vi "FindPosForItem.vi"(0 "reference in":refnum<class "DQMHModuleNode.lvclass">, 1 "SearchItem":string, 2 "AttributesIDs":string[](array[string]), 3 "MethodIDs":string[](array[string]), 5 "error in (no error)":errorcluster) -> (12 "UpperRightPoint":T1 {"y" format="%.2f"; "x" format="%.2f"}, 14 "reference out":refnum<class "DQMHModuleNode.lvclass">, 15 "LeftPoint":T1 {"y" format="%.2f"; "x" format="%.2f"}, 16 "CenterPoint":T1 {"y" format="%.2f"; "x" format="%.2f"}, 17 "RightPoint":T1 {"y" format="%.2f"; "x" format="%.2f"}, 18 "UpperLeftPoint":T1 {"y" format="%.2f"; "x" format="%.2f"}, 19 "error out":errorcluster)   [LabVIEW 2020, in "DQMHModuleNode.lvclass"]
doc: "public void draw(Graphics2D g2, Point2D p, Point2D q)"
uses:
  <resource>/Framework/Providers/Open_GDS/UML/DQMHModuleNode_class/DQMHModuleNode.lvclass
  C:/Program Files (x86)/National Instruments/LabVIEW 2020/resource/Framework/Providers/Open_GDS/UML/RectangularNode_class/RectangularNode.lvclass
  <resource>/Framework/Providers/Open_GDS/UML/General/Point/Point Point2D.ctl
  <resource>/Framework/Providers/Open_GDS/UML/General/Rectangle/Rectangle Rectangle2D.ctl
  <resource>/Framework/Providers/Open_GDS/UML/MultiLineString_class/MultiLineString.lvclass
  <resource>/Framework/Providers/Open_GDS/UML/RectangularNode_class/RectangularNode.lvclass
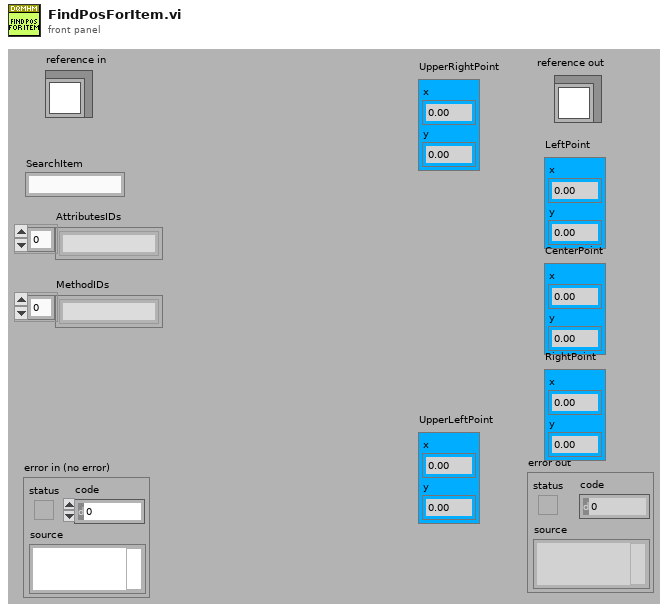
[diagram p1: front panel]
types:
  T1 = typedef "Point Point2D.ctl" = cluster{"x":dbl, "y":dbl}
  T2 = typedef "Rectangle Rectangle2D.ctl" = cluster{"x":dbl, "y":dbl, "width":dbl, "height":dbl}
  T3 = typedef "DQMHModuleNode.lvclass/ObjectAttributes.ctl" = cluster{"DescriptionHeight":dbl, "InternalDataHeight":dbl, "EventsHeight":dbl, "Name":refnum<class "MultiLineString.lvclass">, "Description":refnum<class "MultiLineString.lvclass">, "InternalData":refnum<class "MultiLineString.lvclass">, "Events":refnum<class "MultiLineString.lvclass">, "showDescription":bool, "showInternalData":bool, "showEvents":bool, "DEFAULT_ROUNDING":i32, "DEFAULT_WIDTH":i32, "DEFAULT_HEIGHT":i32, "ClassPath":path, "Template":string, "Icon":u8[][]}
  T4 = typedef "RectangularNode.lvclass/ObjectAttributes.ctl" = cluster{"bounds":T2}
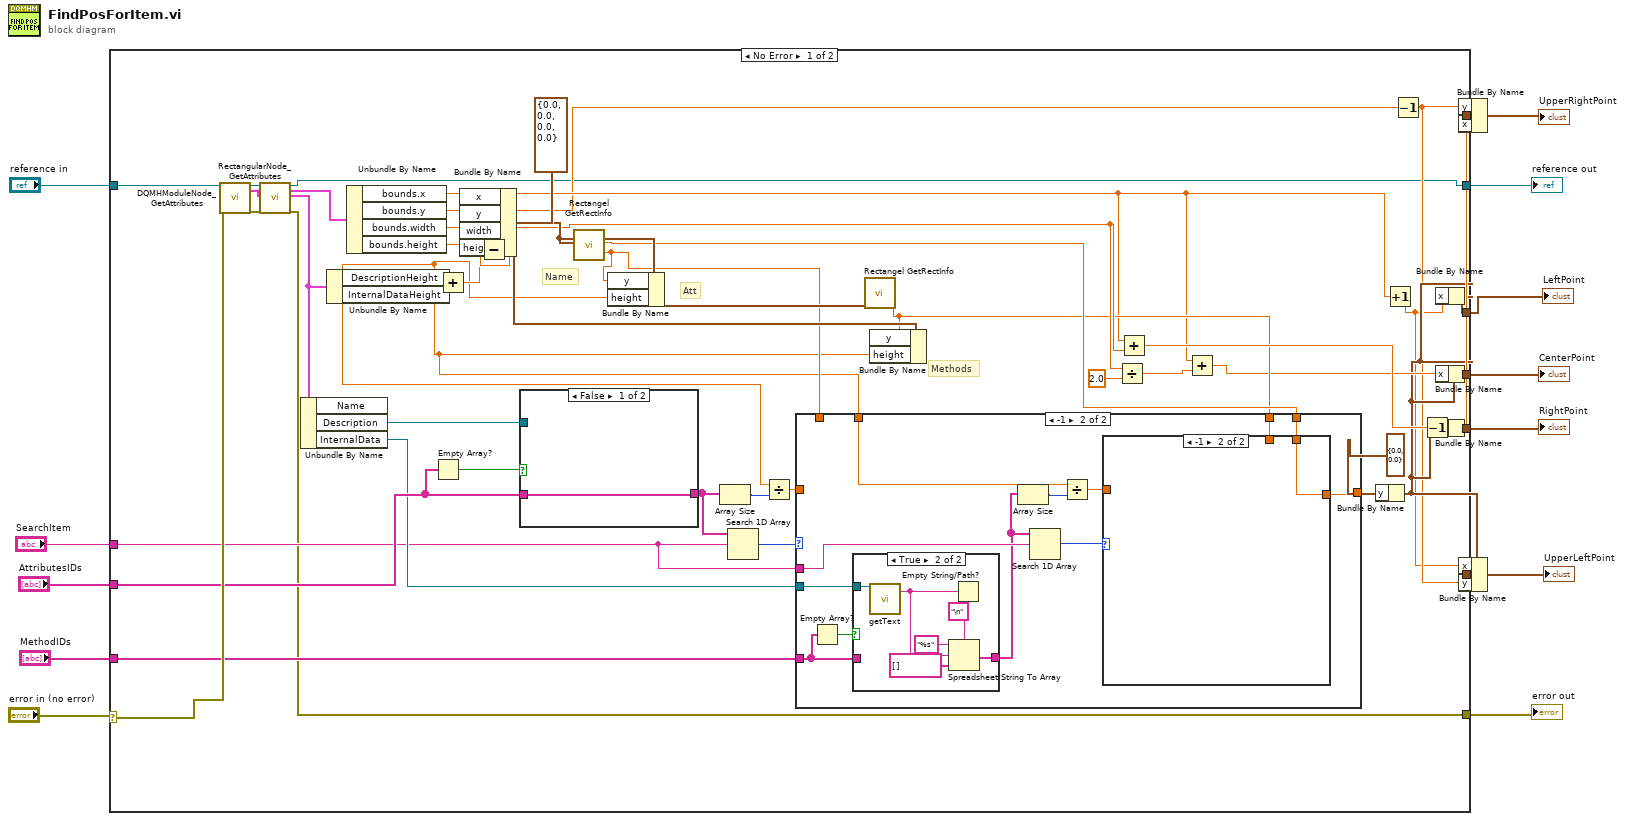
[diagram p0: block diagram]
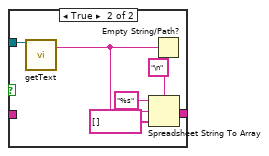
[diagram p2: hidden frame]
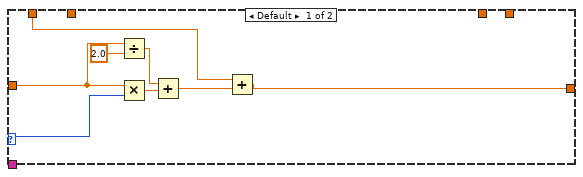
[diagram p3: hidden frame]
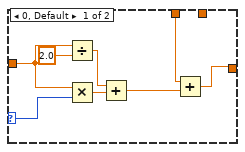
[diagram p4: hidden frame]
diagram:
  n1 = case shown="No Error" "error in (no error)" {
    selector: "error in (no error)" -> [w58 w103]
    tunnel: "reference in" -> [w59 w104]
    tunnel: [w15 w103] -> w11
    tunnel: [w14 w104] -> w10
    tunnel: "SearchItem" -> [w33 _]
    tunnel: "AttributesIDs" -> [w44 _]
    tunnel: [w41 _] -> w6
    tunnel: [w39 _] -> w5
    tunnel: [w38 _] -> w4
    tunnel: "MethodIDs" -> [w35 _]
    tunnel: [w23 _] -> w2
    tunnel: [w21 _] -> w1
    frame No Error {
      # "Methods"
      # "Att"
      # "Name"
      n2 = call <resource>:"DQMHModuleNode_GetAttributes.vi"("reference in"=w59, "error in (no error)"=w58) -> ("reference out"=w17:refnum<class "DQMHModuleNode.lvclass">, "Data"=w18:T3, "error out"=w16:errorcluster)  [unwired: 1 in, 14 out]
      n3 = call <resource>:"RectangularNode_GetAttributes.vi"("reference in"=w17, "error in (no error)"=w16) -> ("reference out"=w14:refnum<class "DQMHModuleNode.lvclass">, "Data"=w13:T4, "error out"=w15:errorcluster)  [unwired: 14 in, 1 out]
      n4 = Unbundle By Name(w18) -> ("Description"=w50:refnum<class "MultiLineString.lvclass">, "InternalData"=w34:refnum<class "MultiLineString.lvclass">)  [unwired: 1 out]
      n5 = Unbundle By Name(w18) -> ("DescriptionHeight"=w48:dbl, "InternalDataHeight"=w29:dbl)
      n6 = Unbundle By Name(w13) -> ("bounds.x"=w28:dbl, "bounds.y"=w24:dbl, "bounds.width"=w37:dbl, "bounds.height"=w56:dbl)
      n7 = Empty Array?(array=w44) -> (empty?=w45:bool)
      n8 = Add(x=w48, y=w29) -> (x+y=w54:dbl)
      n9 = Subtract(x=w56, y=w54) -> (x-y=w55:dbl)
      n10 = Bundle By Name(cluster=T2 {"x"=0.0, "y"=0.0, "width"=0.0, "height"=0.0} ("points"), "x"=w28, "y"=w24, "width"=w37, "height"=w55) -> (w53:T2)
      n11 = case shown="False" w45 {
        tunnel: [w60 w62] -> w51
        tunnel: w50 -> [_ w61]
        tunnel: w44 -> [w60 _]
        frame False {
        }
        frame True {
          n12 = call-dynamic "getText.vi"("reference"=w61) -> ("text"=w63:string)  [unwired: 1 in, 17 out]
          n13 = Spreadsheet String To Array(delimiter (Tab)="\n", format string="%s", spreadsheet string=w63, array type (2D Dbl)=string[] []) -> (array=w62:string[])
          n14 = Empty String/Path?(string/path=w63) -> ()  [unwired: 1 out]
        }
      }
      n15 = call <resource>:"Rectangel GetRectInfo.vi"("bounds"=w53) -> ("centerY"=w31:dbl, "maxY"=w32:dbl)  [unwired: 1 in, 16 out]
      n16 = Bundle By Name(cluster=w53, "y"=w32, "height"=w48) -> (w52:T2)
      n17 = Array Size(array=w51) -> (size(s)=w49:i32)
      n18 = Search 1D Array(1D array=w51, element=w33) -> (index of element=w46:i32)  [unwired: 1 in]
      n19 = Divide(x=w48, y=w49) -> (x/y=w47:dbl)
      n20 = call <resource>:"Rectangel GetRectInfo.vi"("bounds"=w52) -> ("maxY"=w30:dbl)  [unwired: 1 in, 17 out]
      n21 = case shown="-1" w46 {
        selector: w46 -> [w74 _]
        tunnel: w47 -> [w72 _]
        tunnel: [w67 w78] -> w42
        tunnel: w35 -> [_ w85]
        tunnel: w34 -> [_ w84]
        tunnel: w33 -> [_ w82]
        tunnel: w32 -> [w68 _]
        tunnel: w31 -> [_ w79]
        tunnel: w30 -> [_ w77]
        tunnel: w29 -> [_ w76]
        frame Default {
          n22 = Divide(x=w72, y=2.0) -> (x/y=w70:dbl)
          n23 = Multiply(x=w72, y=w74) -> (x*y=w73:dbl)
          n24 = Add(x=w70, y=w73) -> (x+y=w69:dbl)
          n25 = Add(x=w68, y=w69) -> (x+y=w67:dbl)
        }
        frame -1 {
          n26 = Empty Array?(array=w85) -> (empty?=w86:bool)
          n27 = case shown="True" w86 {
            tunnel: [w96 w98] -> w81
            tunnel: w84 -> [_ w97]
            tunnel: w85 -> [w96 _]
            frame False {
            }
            frame True {
              n28 = call-dynamic "getText.vi"("reference"=w97) -> ("text"=w99:string)  [unwired: 1 in, 17 out]
              n29 = Spreadsheet String To Array(delimiter (Tab)="\n", format string="%s", spreadsheet string=w99, array type (2D Dbl)=string[] []) -> (array=w98:string[])
              n30 = Empty String/Path?(string/path=w99) -> ()  [unwired: 1 out]
            }
          }
          n31 = Array Size(array=w81) -> (size(s)=w83:i32)
          n32 = Search 1D Array(1D array=w81, element=w82) -> (index of element=w80:i32)  [unwired: 1 in]
          n33 = Divide(x=w76, y=w83) -> (x/y=w75:dbl)
          n34 = case shown="-1" w80 {
            selector: w80 -> [w87 _]
            tunnel: w79 -> [_ w95]
            tunnel: [w89 w95] -> w78
            tunnel: w77 -> [w90 _]
            tunnel: w75 -> [w88 _]
            frame 0, Default {
              n35 = Divide(x=w88, y=2.0) -> (x/y=w92:dbl)
              n36 = Multiply(x=w88, y=w87) -> (x*y=w94:dbl)
              n37 = Add(x=w92, y=w94) -> (x+y=w91:dbl)
              n38 = Add(x=w90, y=w91) -> (x+y=w89:dbl)
            }
            frame -1 {
            }
          }
        }
      }
      n39 = Bundle By Name(cluster=w53, "y"=w30, "height"=w29) -> ()  [unwired: 1 out]
      n40 = Divide(x=w37, y=2.0) -> (x/y=w27:dbl)
      n41 = Add(x=w28, y=w37) -> (x+y=w36:dbl)
      n42 = Add(x=w28, y=w27) -> (x+y=w26:dbl)
      n43 = Bundle By Name(cluster=T1 {"x"=0.0, "y"=0.0} ("LeftPoint"), "y"=w42) -> (w22:T1)
      n44 = Increment(x=w28) -> (x+1=w19:dbl)
      n45 = Decrement(x=w24) -> (x-1=w20:dbl)
      n46 = Decrement(x=w36) -> (x-1=w25:dbl)
      n47 = Bundle By Name(cluster=w22, "x"=w19) -> (w41:T1)
      n48 = Bundle By Name(cluster=w22, "x"=w26) -> (w39:T1)
      n49 = Bundle By Name(cluster=w22, "x"=w25) -> (w38:T1)
      n50 = Bundle By Name(cluster=w22, "y"=w20, "x"=w25) -> (w23:T1)
      n51 = Bundle By Name(cluster=w22, "x"=w19, "y"=w20) -> (w21:T1)
    }
    frame Error {
    }
  }
  "reference out" <- w10
  "error out" <- w11
  "LeftPoint" <- w6
  "CenterPoint" <- w5
  "RightPoint" <- w4
  "UpperRightPoint" <- w2
  "UpperLeftPoint" <- w1
